vi "Text to UTF-8.vi"(5 "text":string) -> (2 "utf-8 text":string)   [LabVIEW 2020]
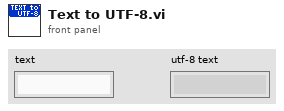
[diagram p1: front panel]
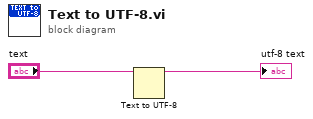
[diagram p0: block diagram]
diagram:
  n1 = Text to UTF-8(11:"text") -> (3:→"utf-8 text":string)  [unwired: 2 in, 1 out]
